vi "Pot Init.vi"(1 "error in":errorcluster) -> (0 "error out":errorcluster)   [LabVIEW 2014]
uses:
  <vilib>/Rock Robotics/SystemInterfaces/AI/FPGA_AIChannel.ctl
  <vilib>/Rock Robotics/SystemInterfaces/Typedef/FPGA_TypedefAnalogModule.ctl
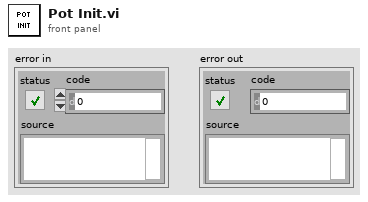
[diagram p1: front panel]
types:
  T1 = typedef "FPGA_AIChannel.ctl" = enum8{"AI 0", "AI 1", "AI 2", "AI 3", "AI MXP 0", "AI MXP 1", "AI MXP 2", "AI MXP 3", "Invalid"}
  T2 = typedef "FPGA_TypedefAnalogModule.ctl" = enum16{"Controller 1"}
  T3 = typedef "WPI_PotentiometerDevRef.ctl" = cluster{"DevStatus":errorcluster, "Controller":T2, "Analog Channel":T1, "Invert Output":bool}
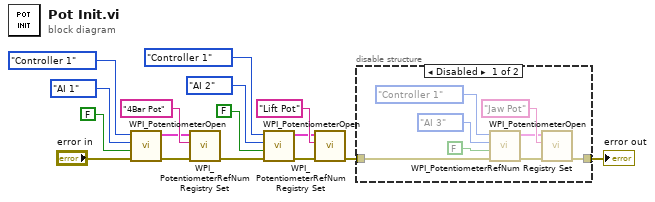
[diagram p0: block diagram]
diagram:
  n1 = call <vilib>:"WPI_PotentiometerOpen.vi"("error in (no error)"="error in", "Invert Output"=FALSE, "Analog Channel"=FPGA_AIChannel."AI 1", "Controller"=FPGA_TypedefAnalogModule."Controller 1") -> ("error out"=w14:errorcluster, "PotDevRef"=w13:T3)  [unwired: 6 in]
  n2 = call <vilib>:"WPI_PotentiometerRefNum Registry Set.vi"("error in (no error)"=w14, "refnum name"="4Bar Pot", "PotDevRef"=w13) -> ("error out"=w9:errorcluster)  [unwired: 7 in, 1 out]
  n3 = call <vilib>:"WPI_PotentiometerOpen.vi"("error in (no error)"=w9, "Invert Output"=FALSE, "Analog Channel"=FPGA_AIChannel."AI 2", "Controller"=FPGA_TypedefAnalogModule."Controller 1") -> ("error out"=w6:errorcluster, "PotDevRef"=w5:T3)  [unwired: 6 in]
  n4 = call <vilib>:"WPI_PotentiometerRefNum Registry Set.vi"("error in (no error)"=w6, "refnum name"="Lift Pot", "PotDevRef"=w5) -> ("error out"=w1:errorcluster)  [unwired: 7 in, 1 out]
  n5 = disable-structure shown="Disabled" {
    disable-tunnel: [w24 w25] -> w8
    disable-tunnel: w1 -> [w23 w25]
    frame Disabled {
      n6 = call <vilib>:"WPI_PotentiometerOpen.vi"("error in (no error)"=w23, "Invert Output"=FALSE, "Analog Channel"=FPGA_AIChannel."AI 3", "Controller"=FPGA_TypedefAnalogModule."Controller 1") -> ("error out"=w21:errorcluster, "PotDevRef"=w20:T3)  [unwired: 6 in]
      n7 = call <vilib>:"WPI_PotentiometerRefNum Registry Set.vi"("error in (no error)"=w21, "refnum name"="Jaw Pot", "PotDevRef"=w20) -> ("error out"=w24:errorcluster)  [unwired: 7 in, 1 out]
    }
    frame Enabled {
    }
  }
  "error out" <- w8
